vi "Add State (to Dictionaries).vi"(8 "error in (no error)":errorcluster, 10 "Routing State":T1, 11 "Channel Ref in":T3 format="%.0x") -> (0 "error out":errorcluster, 3 "Channel Ref out":T3=18446744073709551615 format="%.0x")   [LabVIEW 2017, in "Switch Scripting.lvlib"]
uses:
  Switch Scripting.lvlib
  <vilib>/NI Veristand/Custom Device API/Custom Device Item Ref.ctl
  Routing State.ctl
  Connection.ctl
  NationalInstruments.VeriStand.SystemDefinitionAPI
  Utility/Connection to String.vi
  Shared/Constants.vi
  <vilib>/NI VeriStand/Custom Device API/Custom Device API.lvlib
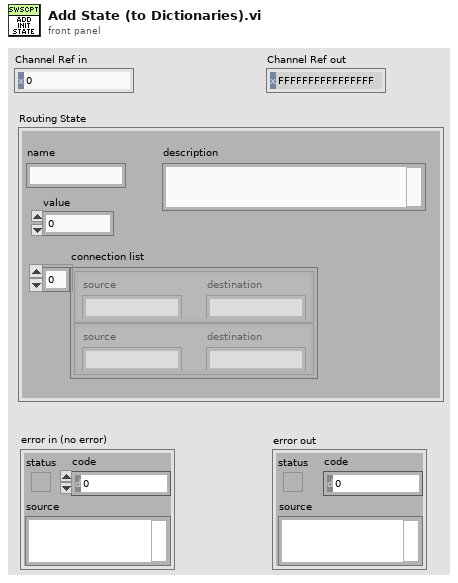
[diagram p1: front panel]
types:
  T1 = typedef "Switch Scripting.lvlib/Routing State.ctl" = cluster{"name":string, "description":string, "value":i32, "connection list":T2[]}
  T2 = typedef "Switch Scripting.lvlib/Connection.ctl" = cluster{"source":string, "destination":string}
  T3 = typedef "Custom Device API.lvlib/Custom Device Item Ref.ctl" = u64
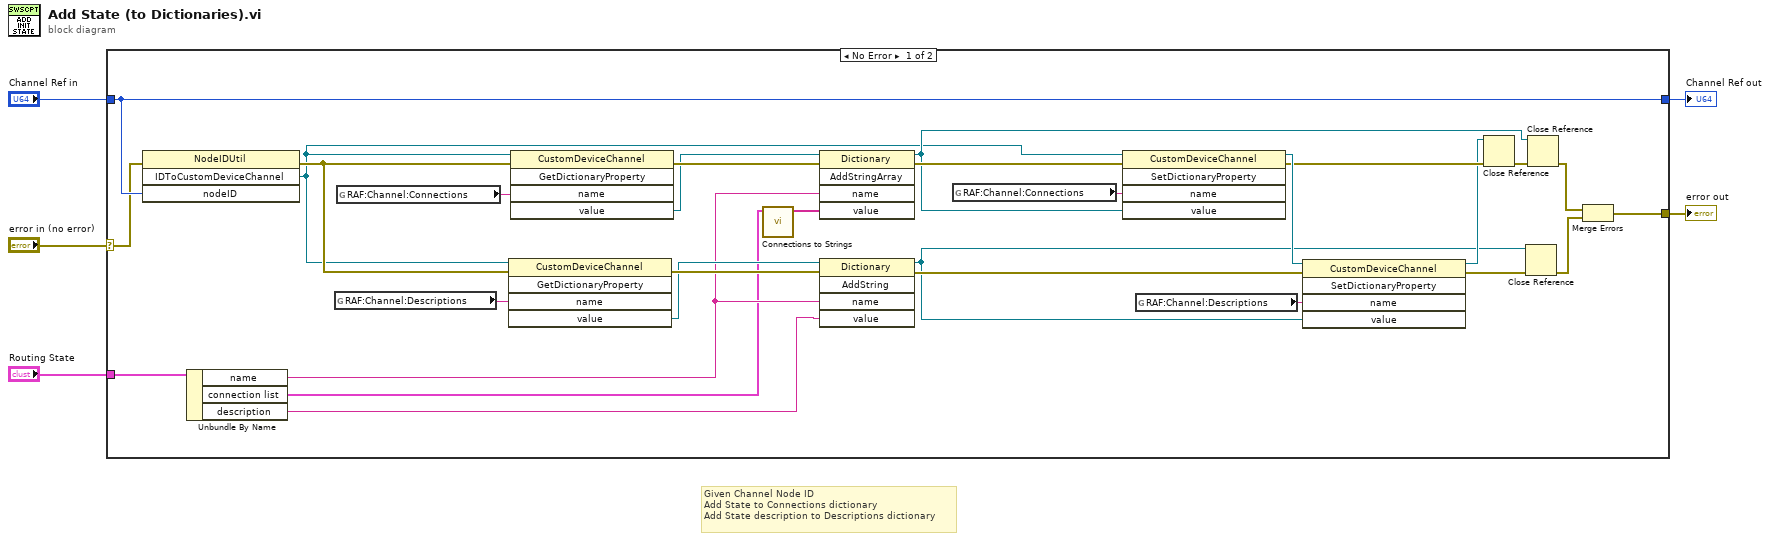
[diagram p0: block diagram]
diagram:
  # "Given Channel Node ID\nAdd State to Connections dictionary\nAdd State description to Descriptions dictionary"
  n1 = case shown="No Error" "error in (no error)" {
    selector: "error in (no error)" -> [w32 w36]
    tunnel: [w12 w36] -> w4
    tunnel: "Channel Ref in" -> [w33 w35]
    tunnel: [w33 w35] -> w2
    tunnel: "Routing State" -> [w10 _]
    frame No Error {
      n2 = invoke class="NodeIDUtil" method="IDToCustomDeviceChannel"(error in=w32, "nodeID"=w33) -> (error out=w23:errorcluster, "IDToCustomDeviceChannel"=w20:refnum<k24>)  [unwired: 2 in, 2 out]
      n3 = Unbundle By Name(w10) -> ("name"=w9:string, "connection list"=w7:T2[], "description"=w6:string)
      n4 = global read "Constants.vi" "RAF:Channel:Descriptions"() -> (w24:string)
      n5 = global read "Constants.vi" "RAF:Channel:Connections"() -> (w29:string)
      n6 = invoke class="CustomDeviceChannel" method="GetDictionaryProperty"(reference=w20, error in=w23, "name"=w24) -> (error out=w22:errorcluster, "value"=w21:refnum<k24>)  [unwired: 2 in, 3 out]
      n7 = invoke class="CustomDeviceChannel" method="GetDictionaryProperty"(reference=w20, error in=w23, "name"=w29) -> (error out=w31:errorcluster, "value"=w11:refnum<k24>)  [unwired: 2 in, 3 out]
      n8 = call "Connections to Strings.vi"("connection list"=w7) -> ("connection strings"=w8:string[])  [unwired: 10 in]
      n9 = invoke class="Dictionary" method="AddStringArray"(reference=w11, error in=w31, "name"=w9, "value"=w8) -> (reference out=w27:refnum<k24>, error out=w30:errorcluster)  [unwired: 1 in, 3 out]
      n10 = invoke class="Dictionary" method="AddString"(reference=w21, error in=w22, "name"=w9, "value"=w6) -> (reference out=w16:refnum<k24>, error out=w25:errorcluster)  [unwired: 1 in, 3 out]
      n11 = global read "Constants.vi" "RAF:Channel:Connections"() -> (w28:string)
      n12 = invoke class="CustomDeviceChannel" method="SetDictionaryProperty"(reference=w20, error in=w30, "name"=w28, "value"=w27) -> (reference out=w19:refnum<k24>, error out=w18:errorcluster)  [unwired: 1 in, 3 out]
      n13 = global read "Constants.vi" "RAF:Channel:Descriptions"() -> (w26:string)
      n14 = invoke class="CustomDeviceChannel" method="SetDictionaryProperty"(reference=w19, error in=w25, "name"=w26, "value"=w16) -> (reference out=w17:refnum<k24>, error out=w15:errorcluster)  [unwired: 1 in, 3 out]
      n15 = Close Reference(reference=w17, error in (no error)=w18) -> (error out=w34:errorcluster)
      n16 = Close Reference(reference=w16, error in (no error)=w15) -> (error out=w13:errorcluster)
      n17 = Close Reference(reference=w27, error in (no error)=w34) -> (error out=w14:errorcluster)
      n18 = Merge Errors(w14, w13) -> (w12:errorcluster)
    }
    frame Error {
    }
  }
  "Channel Ref out" <- w2
  "error out" <- w4
